vi "条件结构坑爹温度计.vi"() -> ()   [LabVIEW 2014]
panel:
  out "暂停按钮 5":bool
  in  "停止 3":bool
  in  "温度配置器 3":cluster{"温度上限(摄氏)":dbl, "摄氏度/华氏度":bool}
  out "温度显示器 3":T1 {"温度计" scale=0.0..100.0}
  out "采集进度 3":u8(slide) scale=0.0..10.0
  in  "开始 4":bool
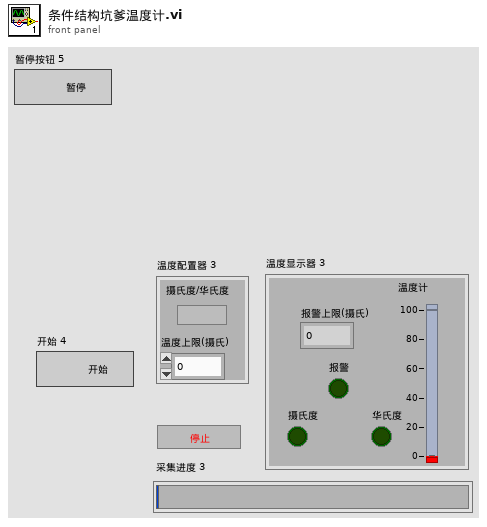
[diagram p1: front panel]
types:
  T1 = cluster{"温度计":dbl, "摄氏度":bool, "报警":bool, "华氏度":bool, "报警上限(摄氏)":dbl}
  T2 = cluster{"温度计":dbl, "摄氏度":bool, "报警":bool, "华氏度":bool, "报警上限":dbl}
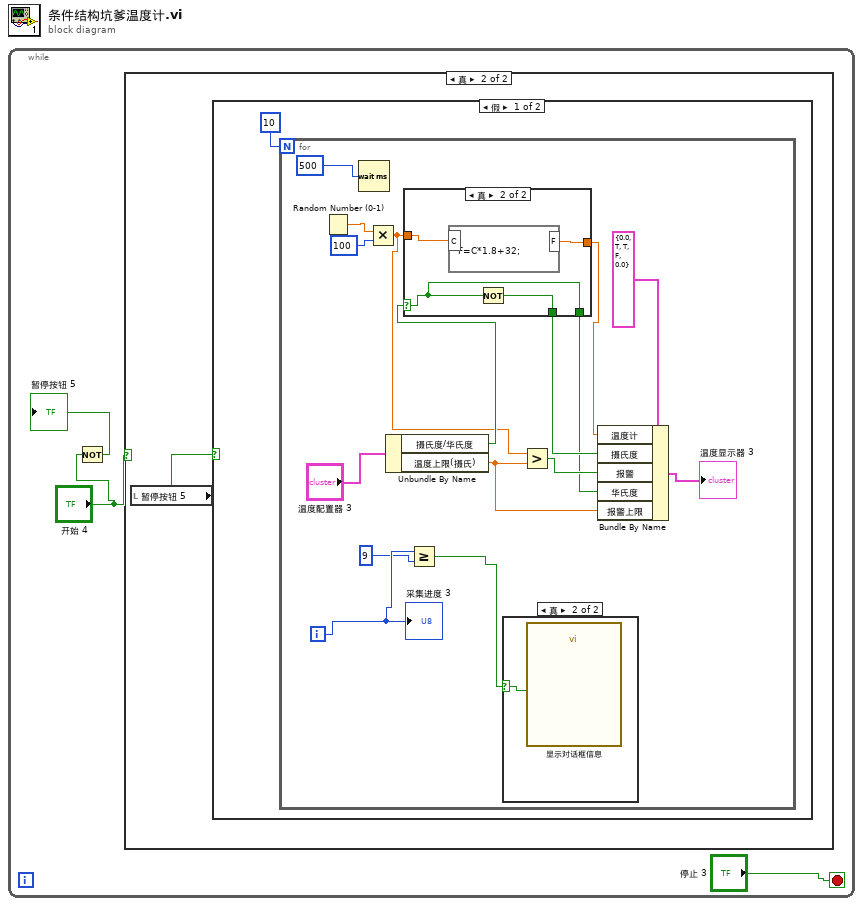
[diagram p0: block diagram]
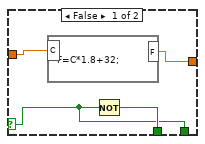
[diagram p4: hidden frame]
diagram:
  n1 = while {
    stop <- "停止 3" stop-if-true
    n2 = Not(x="开始 4") -> (.not. x?=→"暂停按钮 5":bool)
    n3 = case shown="真" "开始 4" {
      frame False {
      }
      frame True {
        n4 = local read "暂停按钮 5"() -> (w4:bool)
        n5 = case shown="假" w4 {
          frame False {
            n6 = for {
              N: 10 -> [_]
              i -> [w9]
              n7 = Random Number (0-1)() -> (number: 0 to 1=w19:dbl)
              n8 = Wait (ms)(milliseconds to wait=500) -> ()  [unwired: 1 out]
              n9 = Multiply(x=w19, y=100) -> (x*y=w15:dbl)
              n10 = Unbundle By Name("温度配置器 3") -> ("摄氏度/华氏度"=w17:bool, "温度上限(摄氏)"=w16:dbl)
              n11 = case shown="真" w17 {
                selector: w17 -> [w23 w29]
                tunnel: w15 -> [w26 w27]
                tunnel: [w24 w30] -> w13
                tunnel: [w23 w29] -> w12
                tunnel: [w25 w28] -> w10
                frame False {
                  n12 = formula code="F=C*1.8+32;"("C"=w26) -> ("F"=w25:dbl)
                  n13 = Not(x=w23) -> (.not. x?=w24:bool)
                }
                frame True {
                  n14 = formula code="F=C*1.8+32;"("C"=w27) -> ("F"=w28:dbl)
                  n15 = Not(x=w29) -> (.not. x?=w30:bool)
                }
              }
              n16 = Greater Or Equal?(x=w9, y=9) -> (x >= y?=w6:bool)
              n17 = case shown="真" w6 {
                selector: w6 -> [_ w22]
                frame False {
                }
                frame True {
                  n18 = call "显示对话框信息"("Enable"=w22) -> ()  [unwired: 9 in, 2 out]
                }
              }
              n19 = Greater?(x=w15, y=w16) -> (0:w14:bool)
              n20 = Bundle By Name(cluster=T2 {"温度计"=0.0, "摄氏度"=TRUE, "报警"=TRUE, "华氏度"=FALSE, "报警上限"=0.0}, "温度计"=w10, "摄氏度"=w13, "报警"=w14, "华氏度"=w12, "报警上限"=w16) -> (→"温度显示器 3":T2)
              "采集进度 3" <- w9
            }
          }
          frame True {
          }
        }
      }
    }
  }
